vi "Auton Drive Dictation.vi"(8 "Reset Encoders":bool, 9 "Distance (inches)":dbl=52.0, 10 "Direction (0-359)":dbl, 11 "Speed (-1 to 1)":dbl=0.75) -> (0 "Joy Y":dbl=0.5124433303800191, 1 "Joy X":dbl, 2 "Distance Reached?":bool)   [LabVIEW 2014]
uses:
  Begin/Global RefNums.vi
  Begin/Global Variables.vi
  <vilib>/Utility/file.llb/Write To Spreadsheet File (I64).vi
  <vilib>/addons/control/pid/NI_PID_pid.lvlib
  <vilib>/addons/control/pid/pid.llb/PID (DBL).vi
panel:
  in  "y":dbl=3.0
  in  "Sigma Conversion":dbl=4.0 format="%#_13g"
  in  "output range":cluster{"output high":dbl, "output low":dbl}={"output high"=1.0, "output low"=-1.0} {"output low" format="%.2f"; "output high" format="%.2f"}
  in  "PID Range":dbl=50.0 format="%#_13g"
  in  "PID gains":T1={"proportional gain (Kc)"=0.01, "integral time (Ti, min)"=0.0, "derivative time (Td, min)"=0.0} {"derivative time (Td, min)" format="%.3f"; "integral time (Ti, min)" format="%.7f"; "proportional gain (Kc)" format="%.3f"}
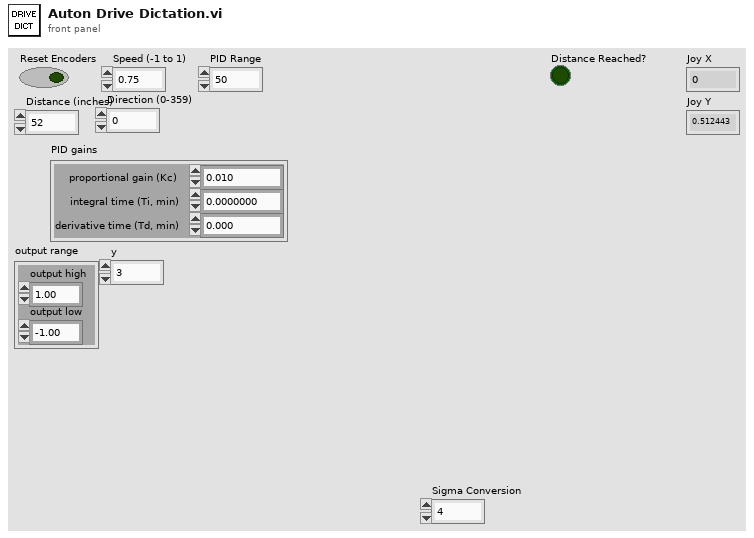
[diagram p1: front panel]
types:
  T1 = cluster{"proportional gain (Kc)":dbl, "integral time (Ti, min)":dbl, "derivative time (Td, min)":dbl}
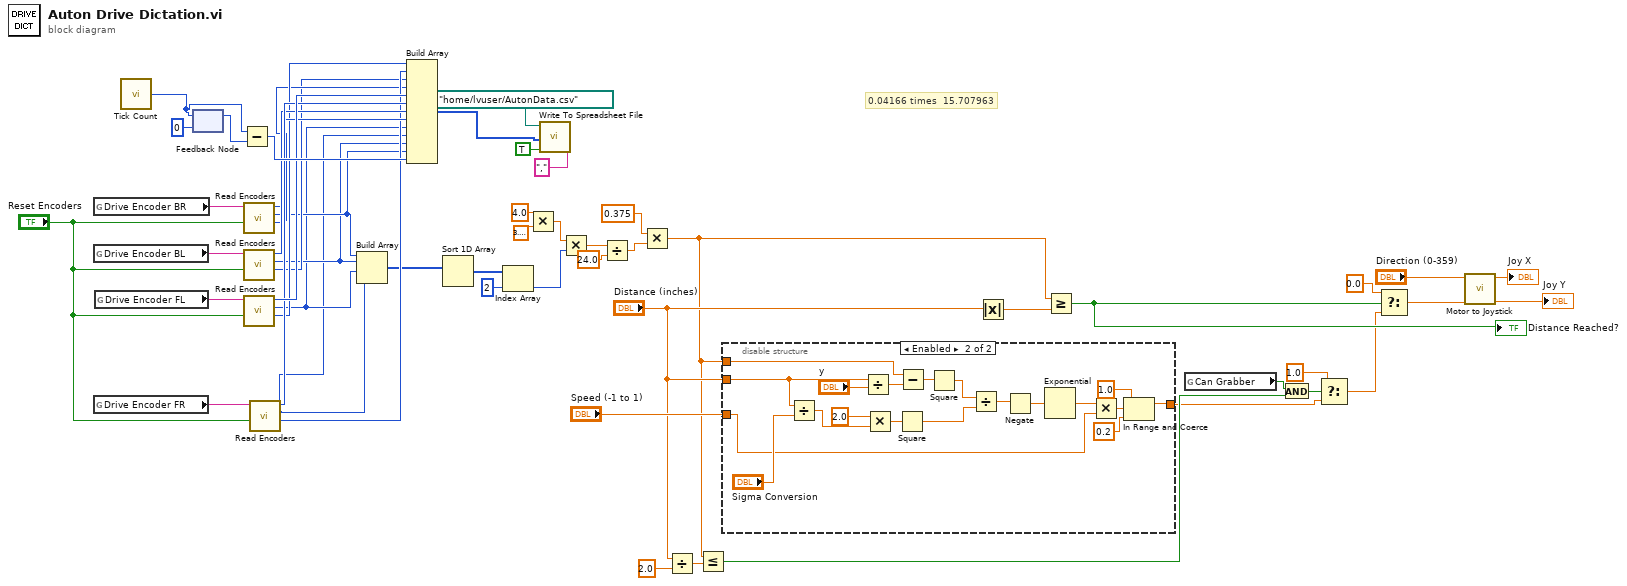
[diagram p0: block diagram]
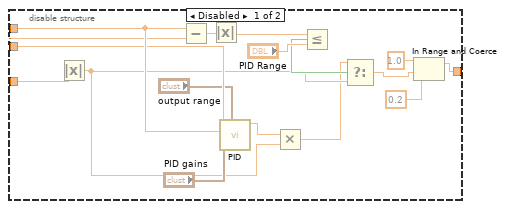
[diagram p2: hidden frame]
diagram:
  # "0.04166 times  15.707963"
  n1 = global read "Global RefNums.vi" "Drive Encoder BR"() -> (w54:string)
  n2 = global read "Global RefNums.vi" "Drive Encoder BL"() -> (w42:string)
  n3 = global read "Global RefNums.vi" "Drive Encoder FR"() -> (w38:string)
  n4 = global read "Global RefNums.vi" "Drive Encoder FL"() -> (w41:string)
  n5 = call "Tick Count"() -> ("Tick Count(mSec)"=w19:u32)
  n6 = feedback-in #1(w19) -> ()
  n7 = feedback #1(u32 0 ("Tick Count(mSec)")) -> (w18:u32)
  n8 = Subtract(x=w19, y=w18) -> (x-y=w20:u32)
  n9 = call "Read Encoders.vi"("Reset Encoders"="Reset Encoders", "Encoder"=w54) -> ("Debug"=w10:i32, "Counts"=w8:i32, "Orig Count"=w13:i32)  [unwired: 7 in]
  n10 = call "Read Encoders.vi"("Reset Encoders"="Reset Encoders", "Encoder"=w42) -> ("Debug"=w9:i32, "Counts"=w7:i32, "Orig Count"=w14:i32)  [unwired: 7 in]
  n11 = call "Read Encoders.vi"("Reset Encoders"="Reset Encoders", "Encoder"=w41) -> ("Debug"=w12:i32, "Counts"=w6:i32, "Orig Count"=w16:i32)  [unwired: 7 in]
  n12 = call "Read Encoders.vi"("Reset Encoders"="Reset Encoders", "Encoder"=w38) -> ("Debug"=w11:i32, "Counts"=w5:i32, "Orig Count"=w15:i32)  [unwired: 7 in]
  n13 = Build Array(w8, w7, w6, w5) -> (w4:i32[])
  n14 = Build Array(w12, w11, w9, w10, w16, w15, w14, w13, w6, w5, w7, w8, w20) -> (w21:u32[])
  n15 = Sort 1D Array(array=w4) -> (sorted array=w3:i32[])
  n16 = Index Array(array=w3, index=2) -> (element=w1:i32)
  n17 = Multiply(x=4.0, y=3.141592653589793) -> (x*y=w47:dbl)
  n18 = call-poly <vilib>:"Write To Spreadsheet File.vi"("delimiter (\\t)"="," ("delimiter (\\t)"), "append to file? (new file:F)"=TRUE, "1D data"=w21, "file path (dialog if empty)"=path "/home/lvuser/AutonData.csv" ("file path (use dialog)")) -> ()  [unwired: 4 in, 1 out]
  n19 = Multiply(x=w47, y=w1) -> (x*y=w46:dbl)
  n20 = Divide(x=w46, y=24.0) -> (x/y=w45:dbl)
  n21 = Multiply(x=0.375 ("y"), y=w45) -> (x*y=w25:dbl)
  n22 = Divide(x="Distance (inches)", y=2.0) -> (x/y=w32:dbl)
  n23 = Less Or Equal?(x=w25, y=w32) -> (x <= y?=w31:bool)
  n24 = disable-structure shown="Enabled" {
    disable-tunnel: w25 -> [w67 w72]
    disable-tunnel: "Distance (inches)" -> [w64 w73]
    disable-tunnel: "Speed (-1 to 1)" -> [w62 w74]
    disable-tunnel: [w55 w75] -> w27
    frame Disabled {
      n25 = Absolute Value(x=w62) -> (abs(x)=w61:dbl)
      n26 = Subtract(x=w67, y=w64) -> (x-y=w69:dbl)
      n27 = Absolute Value(x=w69) -> (abs(x)=w68:dbl)
      n28 = call-poly <vilib>:"PID.vi"("output range"="output range", "PID gains"="PID gains", "process variable"=w67, "setpoint"=w64) -> ("output"=w60:dbl)  [unwired: 6 in, 1 out]
      n29 = Multiply(x=w60, y=w61) -> (x*y=w59:dbl)
      n30 = Less Or Equal?(x=w68, y="PID Range") -> (x <= y?=w65:bool)
      n31 = Select(t=w59, s=w65, f=w61) -> (s? t:f=w56:dbl)
      n32 = In Range and Coerce(upper limit=1.0, x=w56, lower limit=0.2) -> (coerced(x)=w55:dbl)  [unwired: 1 out]
    }
    frame Enabled {
      n33 = Divide(x=w73, y="Sigma Conversion") -> (x/y=w79:dbl)
      n34 = Divide(x=w73, y="y") -> (x/y=w89:dbl)
      n35 = Multiply(x=2.0 ("y"), y=w79) -> (x*y=w86:dbl)
      n36 = Square(x=w86) -> (x^2=w85:dbl)
      n37 = Subtract(x=w72, y=w89) -> (x-y=w88:dbl)
      n38 = Square(x=w88) -> (x^2=w84:dbl)
      n39 = Divide(x=w84, y=w85) -> (x/y=w83:dbl)
      n40 = Negate(x=w83) -> (-x=w82:dbl)
      n41 = Exponential(1:w82) -> (0:w81:dbl)
      n42 = Multiply(x=w81, y=w74) -> (x*y=w78:dbl)
      n43 = In Range and Coerce(upper limit=1.0, x=w78, lower limit=0.2) -> (coerced(x)=w75:dbl)  [unwired: 1 out]
    }
  }
  n44 = Absolute Value(x="Distance (inches)") -> (abs(x)=w43:dbl)
  n45 = Greater Or Equal?(x=w25, y=w43) -> (x >= y?=w53:bool)
  "Distance Reached?" <- w53
  n46 = global read "Global Variables.vi" "Can Grabber"() -> (w30:bool)
  n47 = And(x=w30, y=w31) -> (x .and. y?=w29:bool)
  n48 = Select(t=1.0, s=w29, f=w27) -> (s? t:f=w26:dbl)
  n49 = Select(t=0.0, s=w53, f=w26) -> (s? t:f=w51:dbl)
  n50 = call "Motor to Joystick.vi"("Drive Motor"=w51, "Rotational Motor"="Direction (0-359)") -> ("Joy Y"=→"Joy Y":dbl, "Joy X"=→"Joy X":dbl)  [unwired: 8 in]
